vi "OnOff Read.vi"(9 "error in":errorcluster, 10 "OnOff in":refnum<class "OnOff.lvclass">) -> (0 "OnOff out":refnum<class "OnOff.lvclass">, 1 "OnOff.ACT":bool, 2 "Changed or First Call?":bool, 3 "error out":errorcluster)   [LabVIEW 2023, in "OnOff.lvclass"]
uses:
  OnOff.lvclass
  OnOff.lvclass/OnOff.ctl
  <vilib>/ADAS Replay HIL/Channels/Tag Wrapper/Polymorphic/Read Channel (Boolean).vi
  d71b75cc-87f5-4fee-b6c6-bd8fd19d8a33.vi
  <vilib>/ADAS Replay HIL/Channels/Tag Wrapper/Polymorphic/Read Channel (Boolean).vi/b2f764de-0c1e-4784-a155-687fc995a684.vi
  <vilib>/ADAS Replay HIL/Channels/Tag Wrapper/Polymorphic/Read Channel (Boolean).vi/b2f764de-0c1e-4784-a155-687fc995a684.vi/c28b0ead-42ad-4072-80a2-aca7f2bd7ce3.vi
  <vilib>/ADAS Replay HIL/Channels/Tag Wrapper/Polymorphic/Read Channel (Boolean).vi/b2f764de-0c1e-4784-a155-687fc995a684.vi/219d0231-d98b-4193-b5cc-84f90e3c9091.vi
  <vilib>/ADAS Replay HIL/Channels/Tag Wrapper/Tag Wrapper.lvlib
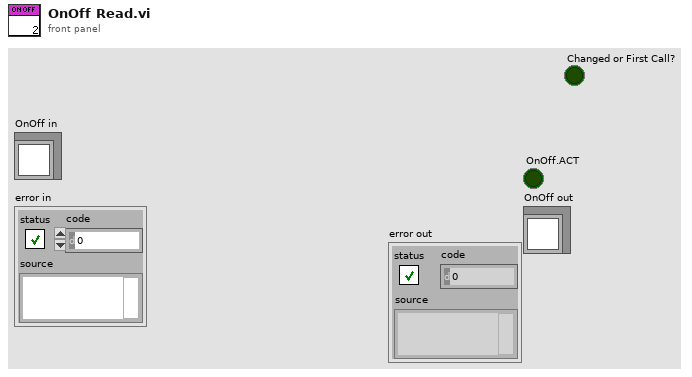
[diagram p1: front panel]
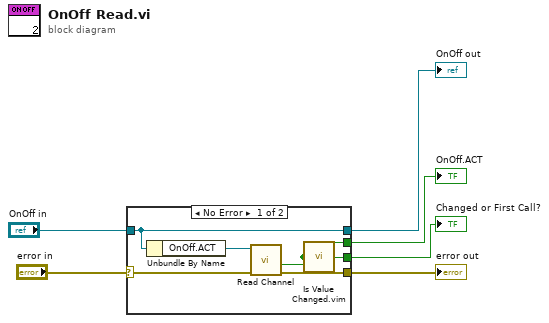
[diagram p0: block diagram]
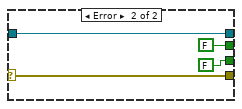
[diagram p2: hidden frame]
diagram:
  n1 = case shown="No Error" "error in" {
    selector: "error in" -> [w11 w16]
    tunnel: [w10 w16] -> w5
    tunnel: [w12 FALSE ("changed or first call?")] -> w4
    tunnel: "OnOff in" -> [w8 w13]
    tunnel: [w9 FALSE] -> w2
    tunnel: [w8 w13] -> w1
    frame No Error {
      n2 = Unbundle By Name(w8) -> ("OnOff.ACT"=w7:refnum<k21>)
      n3 = call-poly <vilib>:"Read Channel.vi"("error in"=w11, "ADAS HIL Channel in"=w7) -> ("error out"=w10:errorcluster, "Timed out?"=w9:bool)  [unwired: 6 in, 2 out]
      n4 = call "Is Value Changed.vim"("value"=w9) -> ("changed or first call?"=w12:bool)
    }
    frame Error {
    }
  }
  "OnOff.ACT" <- w2
  "error out" <- w5
  "Changed or First Call?" <- w4
  "OnOff out" <- w1
